vi "BMcalculate_v2_1.vi"() -> ()   [LabVIEW 2014]
uses:
  <vilib>/Analysis/NI_AALBase.lvlib
  <vilib>/Analysis/baseanly.llb/Mean (DBL).vi
  <vilib>/Analysis/NI_AALPro.lvlib
  <vilib>/Utility/file.llb/Write To Spreadsheet File (DBL).vi
  <vilib>/Utility/file.llb/Read From Spreadsheet File (string).vi
  <vilib>/Analysis/coordinate.llb/2D Cartesian Coordinate Rotation (Array).vi
panel:
  out "path out":path
  in  "(T=X , F=Y)":bool=TRUE
  in  "Filter window size":i32=100
  out "Array":dbl[](array[numeric])
  out "created path 2":path
  out "created path":path
  in  "Save Time-trace":bool
  in  "nm/pixel":dbl=72.5 format="%#_13g"
  in  "Folder path":path
  in  "?":bool
  in  "to":dbl=1.15 format="%#_13g"
  in  "x/y for all":dbl=0.85 format="%#_13g"
  out "filename":string
  in  "Filter mode":T1(ring)=enum."Median_slide window"
  in  "Save to vertical data ?":bool
  in  "?":enum32{"slide by slide", "delay"}(tab)=enum."delay"
  in  "?":bool
  in  "seconds to wait":u32
  in  "?":dbl=7.963 format="%#_13g"
  in  "?":dbl=48.61 format="%#_13g"
  in  "Save BM":bool
  in  "?":bool=TRUE
  in  "Save X-Y plot":bool
  in  "less than":dbl=0.2 format="%#_13g"
  in  "?":bool
  in  "?":bool
  in  "?":bool=TRUE
  in  "?":T2(tab)
  out "Filenames":string[](array[string])
  out "useful AOIs":i32[](array[numeric])
  out "# of AOI":i32[](array[numeric])
  out "% of useful AOIs":dbl
  out "tt # of AOIs":i32
  out "# of Frames":dbl[](array[numeric])
  out "tt # 0f useful AOIs":i32
  out "?":T3(graph)
  out "size(s)":i32
  out "X-Y plot":cluster{dbl[], dbl[]}(graph)
  out "Xstd":dbl
  out "ystd":dbl[](array[numeric])
  out "X":dbl format="%0.2f"
  out "Y":dbl format="%0.2f"
  out "?":T3(graph)
  out "tt # of useful AOIs":i32
  out "xstd":dbl[](array[numeric])
  out "# of AOI":i32
  out "y 2":dbl[](array[numeric])
  out "# of frames":dbl
  out "all y position (pixel)":dbl[][](array[numeric])
  out "all x position (pixel)":dbl[][](array[numeric])
  out "y":dbl[](array[numeric])
  out "x":dbl[](array[numeric])
  out "y":dbl[](array[numeric])
  out "x":dbl[](array[numeric])
  out "number":dbl[][](array[numeric])
  out "all rows":string[][](array[string])
  out "Useful aoi number":string[][](array[string])
  in  "Tab Control":enum32{"Time trace"}(tab)
  out "Time trace":T4(graph)
  in  "Highlight":dbl=30.0
  in  "±":dbl=30.0
  out "aoi":string
  in  "stop frame1":dbl
  in  "start frame1":dbl
  in  "start frame3":dbl
  in  "stop frame2":dbl
  in  "stop frame3":dbl
  in  "start frame2":dbl
  # "Critiria"
  # "±"
  # "nm"
  # "for ssDNA strande exchange \n                    23.776±6.613 nm"
  # "for D-loop  (90+4)\n                    48.61±7.963 nm"
  # "for D-loop  (150+4)\n                    49.57±8.56 nm"
  # "nm"
  # "Buffer wash"
  # "to"
  # "to"
  # "to"
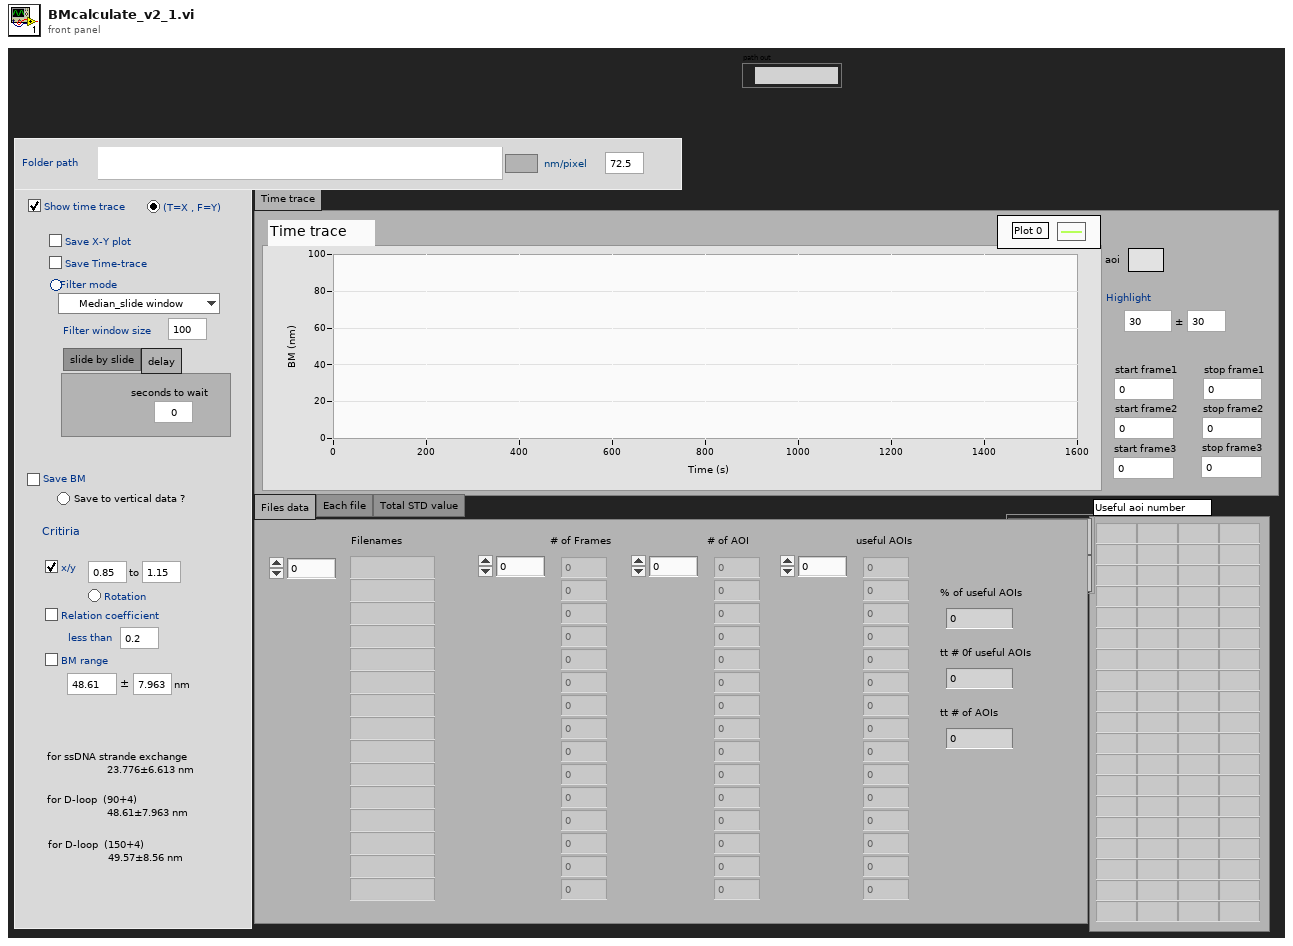
[diagram p1: front panel]
types:
  T1 = enum16{"Median_fix window", "Average_fix window", "Median_slide window", "Average_slide window"}
  T2 = enum32{"Files data", "Each file", "Total STD value"}
  T3 = cluster{"X Values":dbl[], "Histogram: h(x)":i32[]}
  T4 = cluster{"Filtered X":dbl[], "Filtered X":dbl[]}[]
  T5 = cluster{"all y position (pixel)":dbl[], "all x position (pixel)":dbl[]}
  T6 = cluster{"all x position (pixel)":dbl[], "all y position (pixel)":dbl[]}
  T7 = typedef "imagedata.ctl" = cluster{"image type":i32, "image depth":i32, "image":u8[], "mask":u8[], "colors":u32[], "Rectangle":cluster{"left":i16, "top":i16, "right":i16, "bottom":i16}}
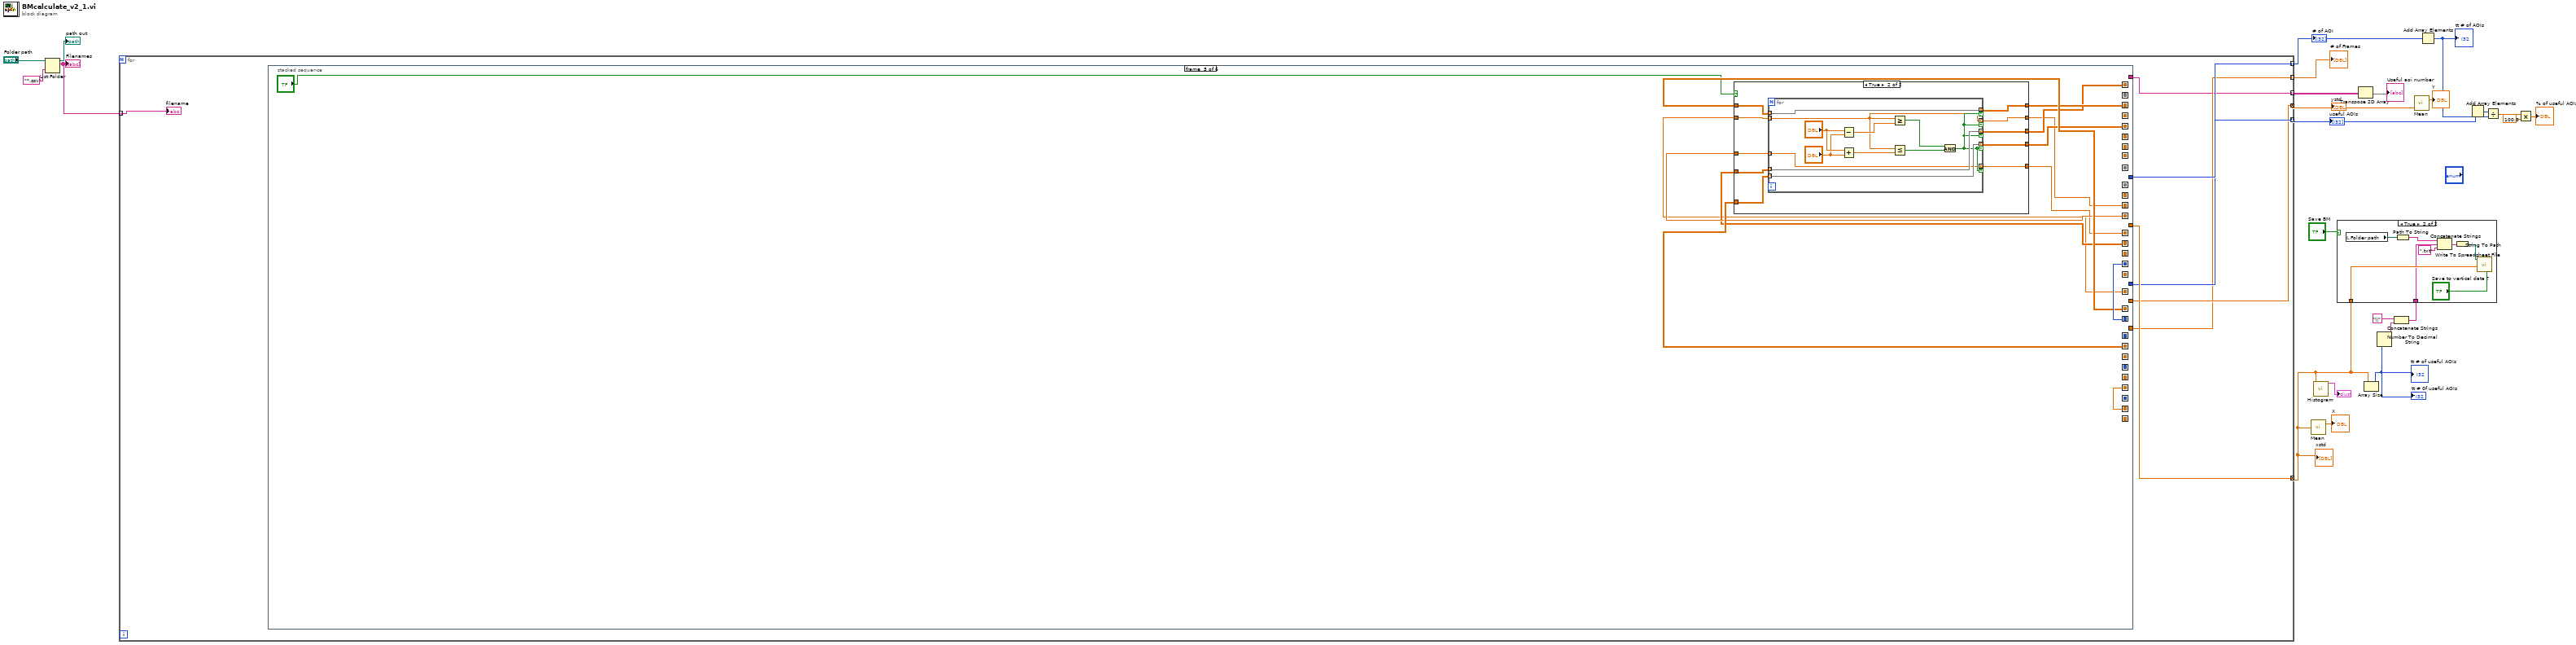
[diagram p0: block diagram]
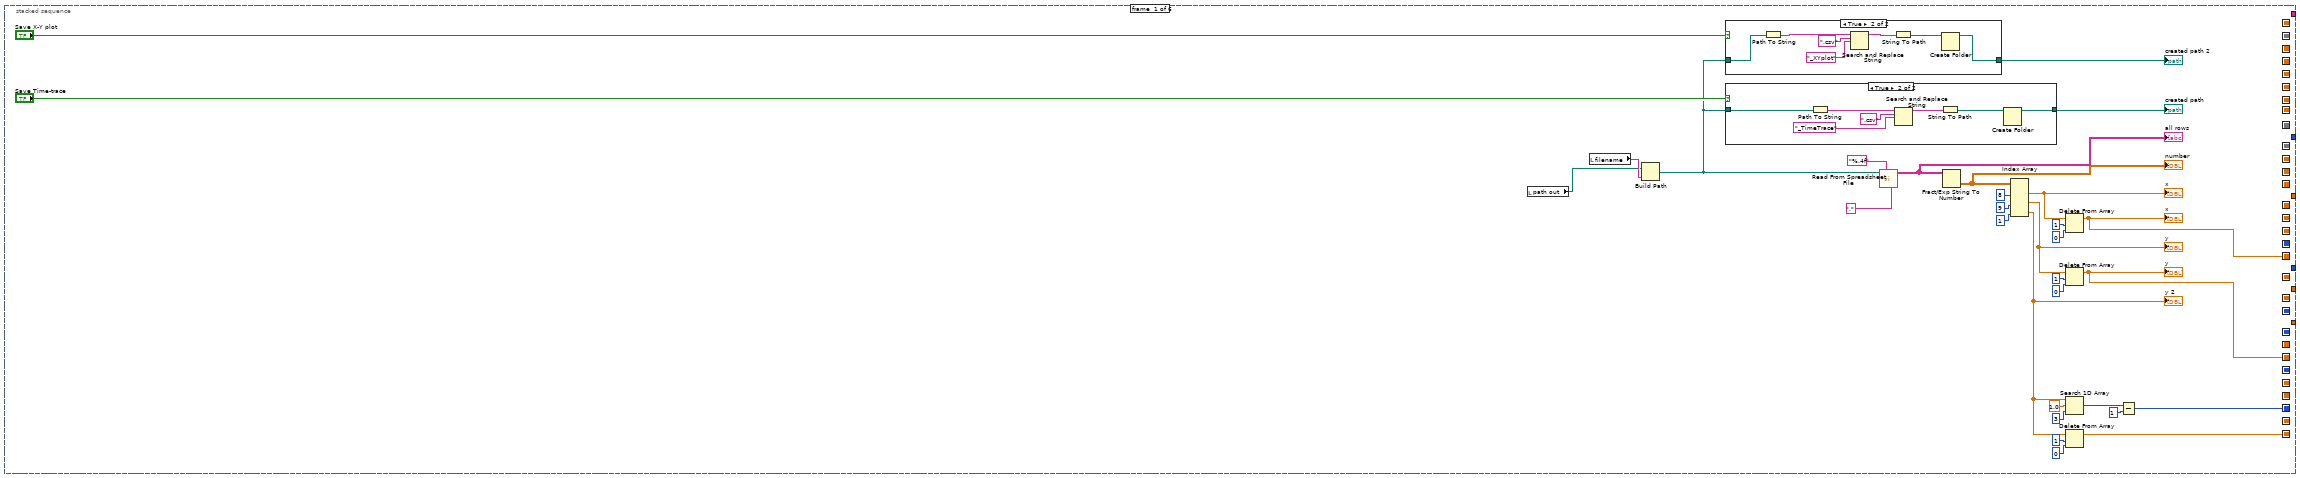
[diagram p3: hidden frame]
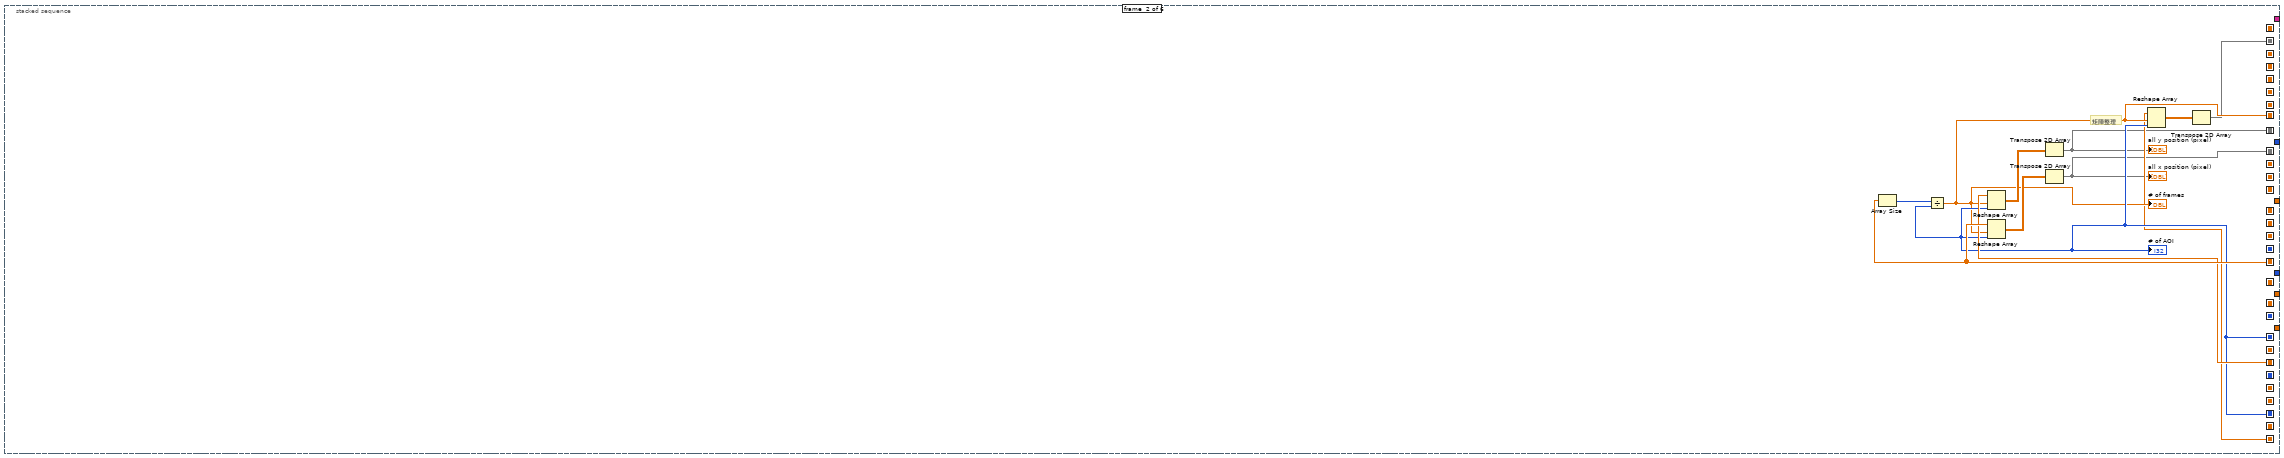
[diagram p6: hidden frame]
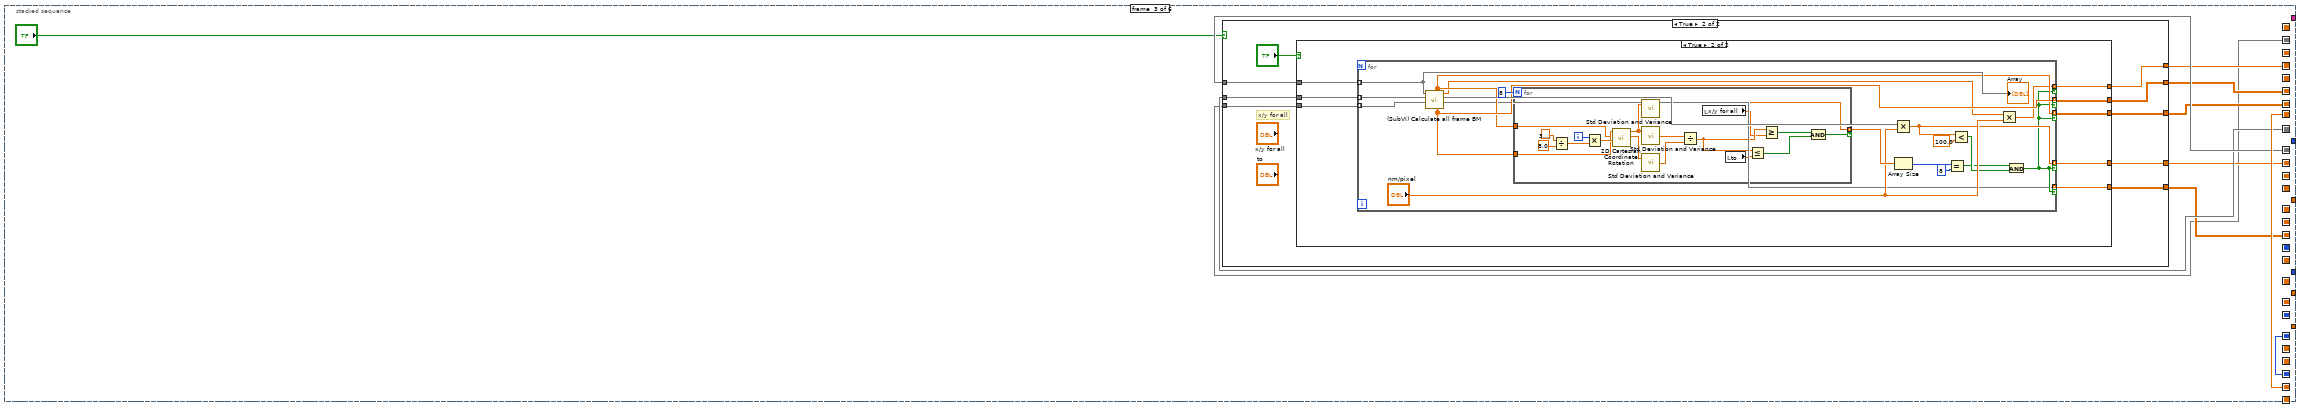
[diagram p7: hidden frame]
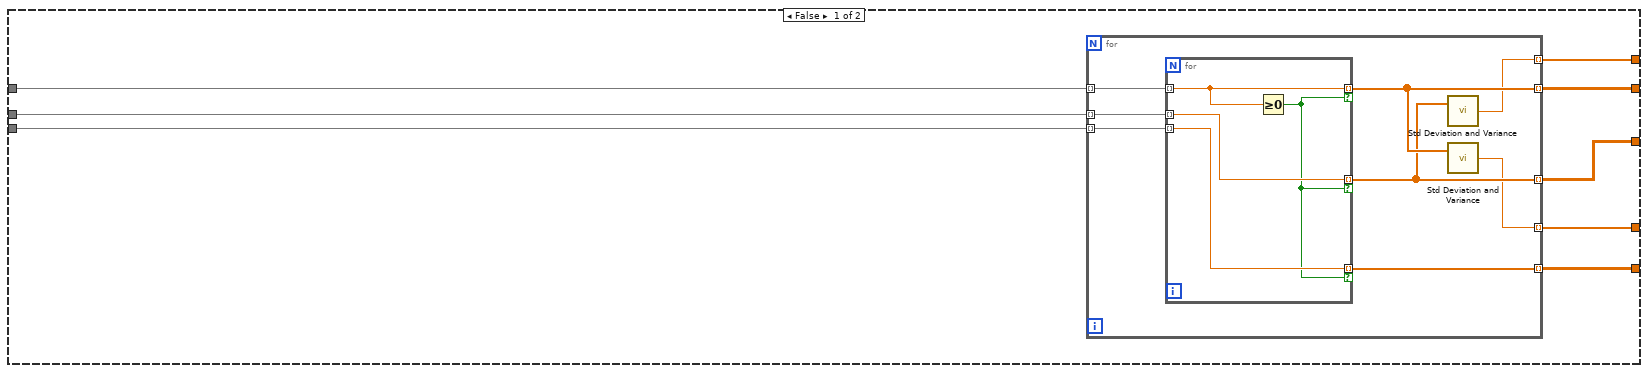
[diagram p8: hidden frame]
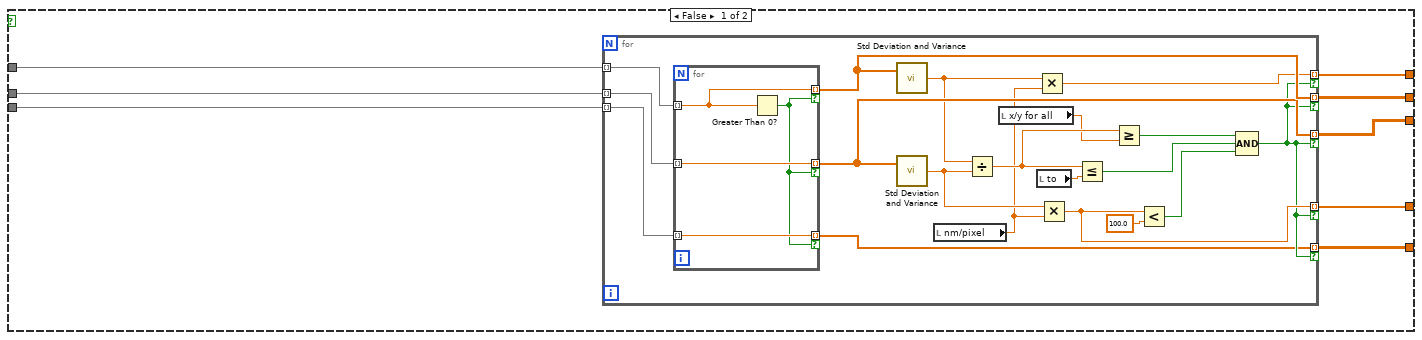
[diagram p9: hidden frame]
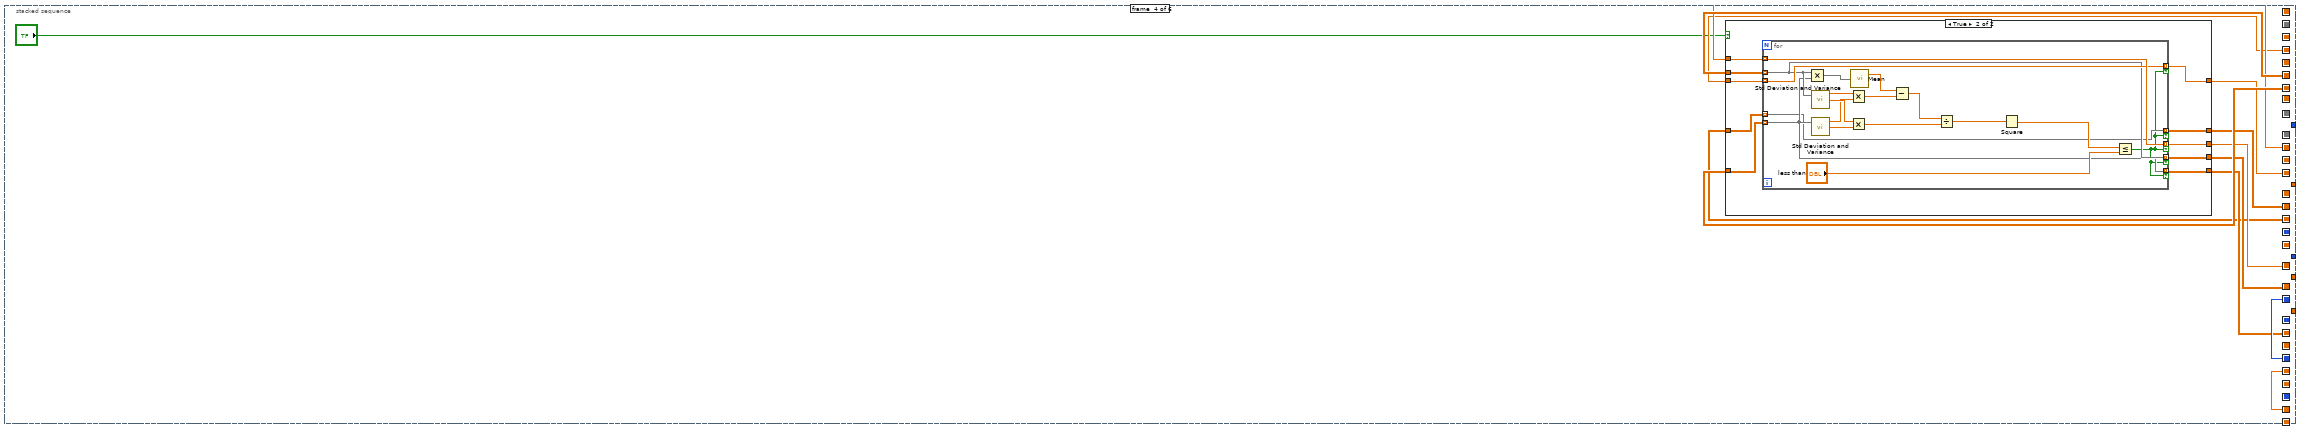
[diagram p10: hidden frame]
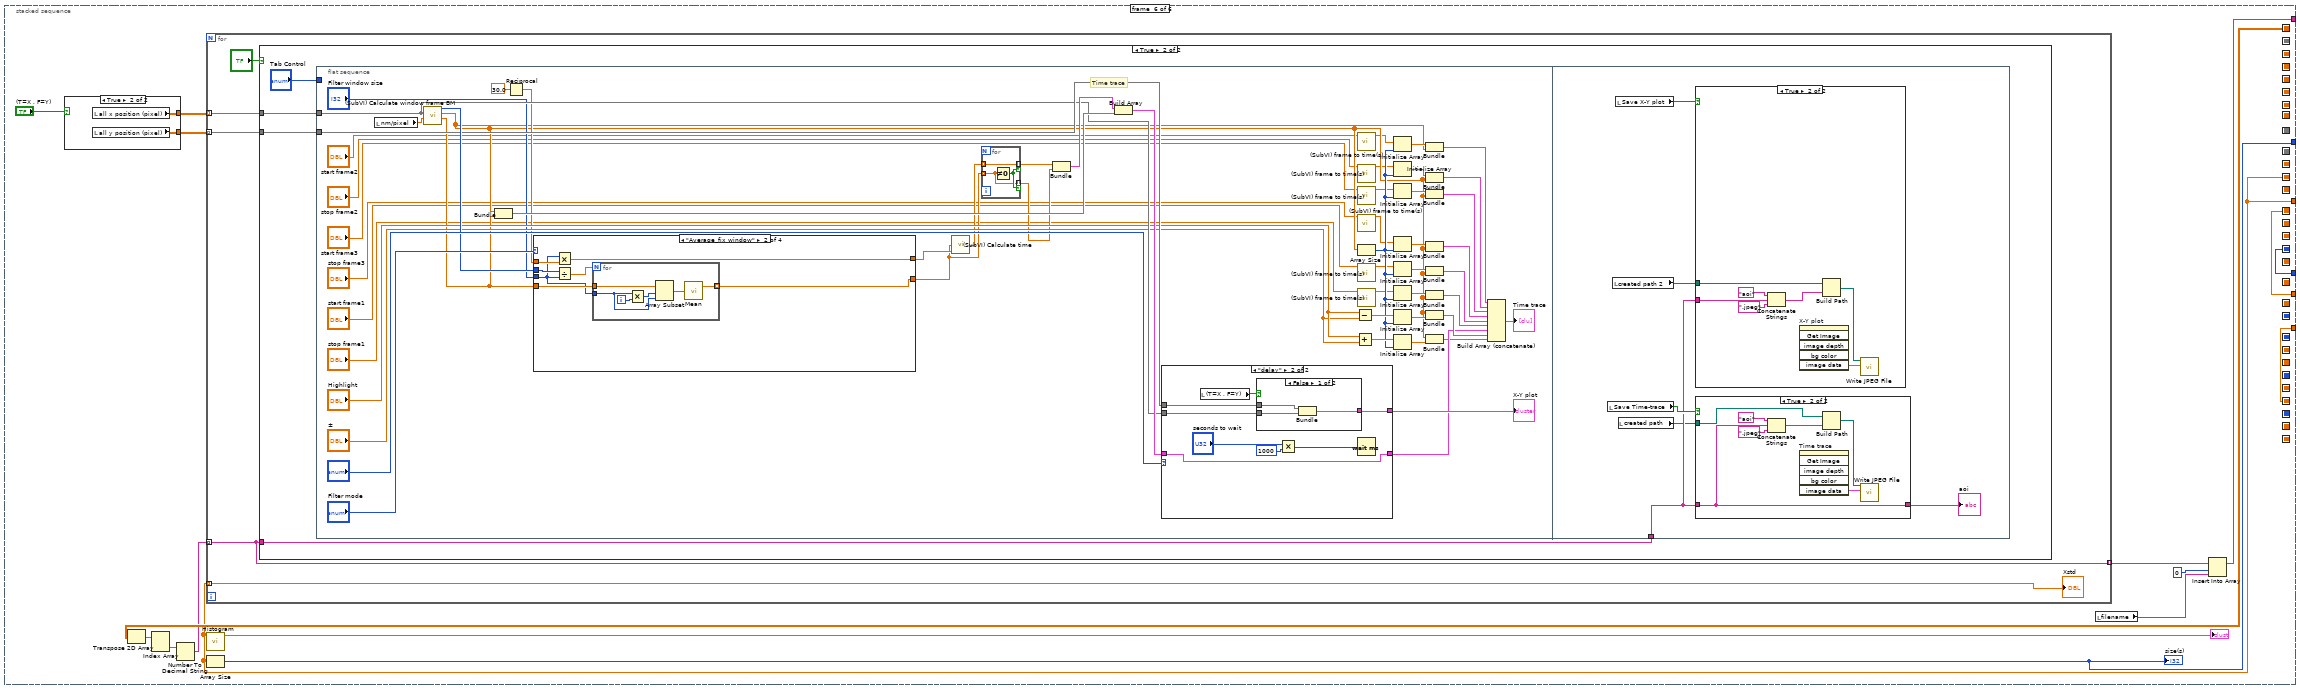
[diagram p13: hidden frame]
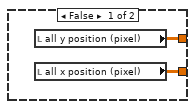
[diagram p14: hidden frame]
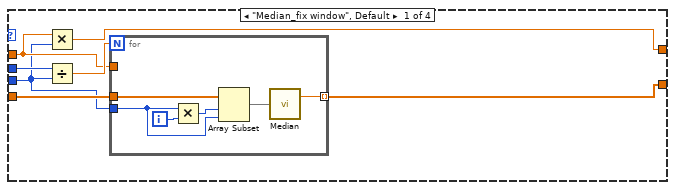
[diagram p16: hidden frame]
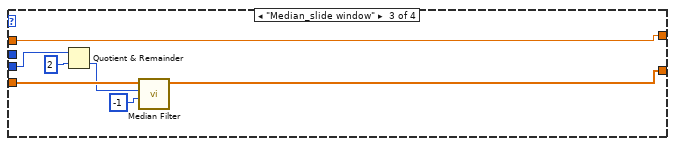
[diagram p17: hidden frame]
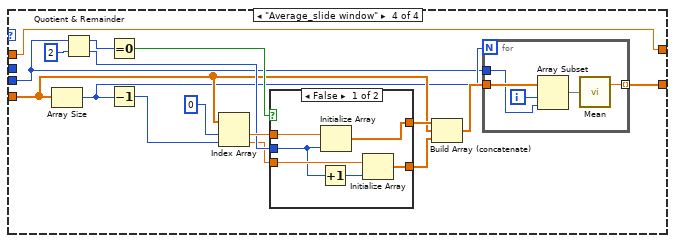
[diagram p18: hidden frame]
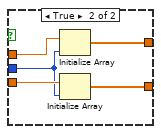
[diagram p19: hidden frame]
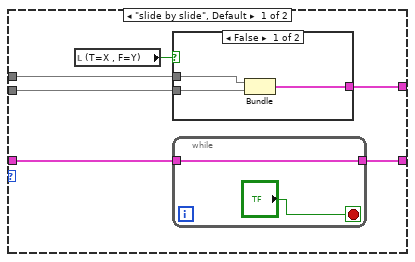
[diagram p20: hidden frame]
diagram:
  n1 = List Folder(path="Folder path", pattern="*.csv") -> (path out=→"path out":path, filenames=w1:string[])  [unwired: 2 in, 2 out]
  "Filenames" <- w1
  n2 = for {
    tunnel: [w31] -> w2 mode=concatenating
    tunnel: [w30] -> w21 mode=indexing
    tunnel: [w29] -> w20 mode=indexing
    tunnel: [w28] -> w12 mode=concatenating
    tunnel: [w27] -> w13 mode=indexing
    tunnel: [w26] -> w4 mode=indexing
    tunnel: w1 -> [w25] mode=indexing
    n3 = stacked-sequence {
      seq-local: [w51 _ _ _ _ _] -> [_ w87 _ _ _ _]
      seq-local: [w50 _ _ _ _ _] -> [_ w86 _ _ _ _]
      seq-local: [w44 _ _ _ _ _] -> [_ w85 _ _ _ _]
      seq-local: [w40 _ _ _ _ _] -> [_ w83 _ _ _ _]
      seq-local: [_ w84 _ _ _ _] -> [_ _ w101 _ _ _]
      seq-local: [_ w85 _ _ _ _] -> [_ _ w100 _ _ _]
      seq-local: [_ w80 _ _ _ _] -> [_ _ w99 _ _ _]
      seq-local: [_ w79 _ _ _ _] -> [_ _ w98 _ _ _]
      seq-local: [_ w81 _ _ _ _] -> [_ _ w91 _ _ _]
      seq-local: [_ _ w100 _ _ _] -> [_ _ _ w219 _ _]
      seq-local: [_ _ w101 _ _ _] -> [_ _ _ w218 _ _]
      seq-local: [_ _ w96 _ _ _] -> [_ _ _ w214 _ _]
      seq-local: [_ _ w95 _ _ _] -> [_ _ _ w217 _ _]
      seq-local: [_ _ w94 _ _ _] -> [_ _ _ w216 _ _]
      seq-local: [_ _ w93 _ _ _] -> [_ _ _ w215 _ _]
      seq-local: [_ _ w92 _ _ _] -> [_ _ _ w208 _ _]
      seq-local: [_ _ _ w219 _ _] -> [_ _ _ _ w265 _]
      seq-local: [_ _ _ w218 _ _] -> [_ _ _ _ w264 _]
      seq-local: [_ _ _ w209 _ _] -> [_ _ _ _ w259 _]
      seq-local: [_ _ _ w212 _ _] -> [_ _ _ _ w263 _]
      seq-local: [_ _ _ w211 _ _] -> [_ _ _ _ w261 _]
      seq-local: [_ _ _ w210 _ _] -> [_ _ _ _ w254 _]
      seq-local: [_ _ _ w207 _ _] -> [_ _ _ _ w256 _]
      seq-local: [_ _ _ _ w265 _] -> [_ _ _ _ _ w311]
      seq-local: [_ _ _ _ w264 _] -> [_ _ _ _ _ w310]
      seq-local: [_ _ _ _ w258 _] -> [_ _ _ _ _ w309]
      seq-local: [_ _ _ _ w262 _] -> [_ _ _ _ _ _]
      seq-local: [_ _ _ _ w260 _] -> [_ _ _ _ _ _]
      seq-local: [_ _ _ _ w253 _] -> [_ _ _ _ _ w302]
      seq-local: [_ _ _ _ w255 _] -> [_ _ _ _ _ w306]
      tunnel: [_ _ _ _ _ w302] -> w31
      tunnel: [_ _ _ _ _ w307] -> w30
      tunnel: [_ _ _ _ _ w311] -> w29
      tunnel: [_ _ _ _ _ w310] -> w27
      tunnel: [_ _ _ _ _ w309] -> w28
      tunnel: [_ _ _ _ _ w298] -> w26
      frame #0 {
        n4 = local read "path out"() -> (w32:path)
        n5 = local read "filename"() -> (w33:string)
        n6 = Build Path(base path=w32, name or relative path=w33) -> (appended path=w35:path)
        n7 = case shown="True" "Save X-Y plot" {
          tunnel: w35 -> [w71 w78]
          tunnel: [w71 w72] -> w39
          frame False {
          }
          frame True {
            n8 = Path To String(path=w78) -> (string=w77:string)
            n9 = Search and Replace String(input string=w77, search string=".csv", replace string="_XYplot" ("replace string (\"\")")) -> (result string=w74:string)  [unwired: 5 in, 3 out]
            n10 = String To Path(string=w74) -> (path=w73:path)
            n11 = Create Folder(path (use dialog)=w73) -> (created path=w72:path)  [unwired: 2 in, 2 out]
          }
        }
        "created path 2" <- w39
        n12 = case shown="True" "Save Time-trace" {
          tunnel: w35 -> [w63 w70]
          tunnel: [w63 w64] -> w34
          frame False {
          }
          frame True {
            n13 = Path To String(path=w70) -> (string=w69:string)
            n14 = Search and Replace String(input string=w69, search string=".csv", replace string="_TimeTrace" ("replace string (\"\")")) -> (result string=w66:string)  [unwired: 5 in, 3 out]
            n15 = String To Path(string=w66) -> (path=w65:path)
            n16 = Create Folder(path (use dialog)=w65) -> (created path=w64:path)  [unwired: 2 in, 2 out]
          }
        }
        "created path" <- w34
        n17 = call-poly <vilib>:"Read From Spreadsheet File.vi"("delimiter (\\t)"="," ("delimiter (\\t)"), "format (%s)"="%.4f" ("format (%.3f)"), "file path (dialog if empty)"=w35) -> ("all rows"=w61:string[][])  [unwired: 4 in, 4 out]
        "all rows" <- w61
        n18 = Fract/Exp String To Number(string=w61) -> (number=w60:dbl[][])  [unwired: 3 in, 1 out]
        "number" <- w60
        n19 = Index Array(array=w60, index (col) #1=8 ("disabled index (col)"), index (col) #2=9 ("index (col)"), index (col) #3=1 ("index (col)")) -> (element #1=w52:dbl[], element #2=w53:dbl[], element #3=w41:dbl[])  [unwired: 3 in]
        "x" <- w52
        "y" <- w53
        "y 2" <- w41
        n20 = Delete From Array(array=w52, length=1, index=0) -> (array with subset deleted=w51:dbl[])  [unwired: 1 out]
        "x" <- w51
        n21 = Delete From Array(array=w53, length=1, index=0) -> (array with subset deleted=w50:dbl[])  [unwired: 1 out]
        "y" <- w50
        n22 = Search 1D Array(1D array=w41, element=1.0, start index (0)=3) -> (index of element=w46:i32)
        n23 = Delete From Array(array=w41, length=1, index=0) -> (array with subset deleted=w40:dbl[])  [unwired: 1 out]
        n24 = Subtract(x=w46, y=1) -> (x-y=w44:i32)
      }
      frame #1 {
        # "矩陣整理"
        n25 = Array Size(array=w87) -> (size(s)=w88:i32)
        n26 = Divide(x=w88, y=w85) -> (x/y=w84:dbl)
        "# of frames" <- w84
        n27 = Reshape Array(w86, w84, w85) -> (w90:dbl[][])
        n28 = Reshape Array(w87, w84, w85) -> (w89:dbl[][])
        n29 = Transpose 2D Array(2D array=w90) -> (transposed array=w79:dbl[][])
        "all y position (pixel)" <- w79
        n30 = Transpose 2D Array(2D array=w89) -> (transposed array=w80:dbl[][])
        "all x position (pixel)" <- w80
        n31 = Reshape Array(w83, w84, w85) -> (w82:dbl[][])
        n32 = Transpose 2D Array(2D array=w82) -> (transposed array=w81:dbl[][])
        "# of AOI" <- w85
      }
      frame #2 {
        n33 = case shown="True" "?" {
          tunnel: [w107 w130] -> w95
          tunnel: [w106 w129] -> w94
          tunnel: w99 -> [w109 w128]
          tunnel: w98 -> [w108 w127]
          tunnel: [w105 w126] -> w93
          tunnel: [w104 w125] -> w96
          tunnel: w91 -> [w103 w123]
          tunnel: [w102 w122] -> w92
          frame False {
            n34 = for {
              tunnel: w109 -> [w117] mode=indexing
              tunnel: w108 -> [w116] mode=indexing
              tunnel: [w115] -> w107 mode=indexing
              tunnel: [w114] -> w106 mode=indexing
              tunnel: [w113] -> w105 mode=indexing
              tunnel: [w112] -> w104 mode=indexing
              tunnel: w103 -> [w111] mode=indexing
              tunnel: [w110] -> w102 mode=indexing
              n35 = for {
                tunnel: w117 -> [w120] mode=indexing
                tunnel: w116 -> [w121] mode=indexing
                tunnel: [w120] -> w115 mode=indexing if=w118
                tunnel: [w121] -> w114 mode=indexing if=w118
                tunnel: w111 -> [w119] mode=indexing
                tunnel: [w119] -> w110 mode=indexing if=w118
                n36 = Greater Or Equal To 0?(x=w120) -> (x >= 0?=w118:bool)
              }
              n37 = call <vilib>:"Std Deviation and Variance.vi"("X"=w114) -> ("standard deviation"=w112:dbl)  [unwired: 1 in, 2 out]
              n38 = call <vilib>:"Std Deviation and Variance.vi"("X"=w115) -> ("standard deviation"=w113:dbl)  [unwired: 1 in, 2 out]
            }
          }
          frame True {
            # "x/y for all"
            n39 = case shown="True" "?" {
              tunnel: w127 -> [w137 w169]
              tunnel: w128 -> [w138 w168]
              tunnel: [w136 w167] -> w130
              tunnel: [w135 w166] -> w129
              tunnel: [w134 w165] -> w126
              tunnel: [w133 w164] -> w125
              tunnel: w123 -> [w132 w163]
              tunnel: [w131 w162] -> w122
              frame False {
                n40 = for {
                  tunnel: w138 -> [w157] mode=indexing
                  tunnel: w137 -> [w156] mode=indexing
                  tunnel: [w155] -> w136 mode=indexing if=w142
                  tunnel: [w154] -> w135 mode=indexing if=w142
                  tunnel: [w143] -> w134 mode=indexing if=w142
                  tunnel: [w146] -> w133 mode=indexing if=w142
                  tunnel: [w140] -> w131 mode=indexing if=w142
                  tunnel: w132 -> [w141] mode=indexing
                  n41 = for {
                    tunnel: w157 -> [w160] mode=indexing
                    tunnel: w156 -> [w161] mode=indexing
                    tunnel: [w160] -> w155 mode=indexing if=w158
                    tunnel: [w161] -> w154 mode=indexing if=w158
                    tunnel: w141 -> [w159] mode=indexing
                    tunnel: [w159] -> w140 mode=indexing if=w158
                    n42 = Greater Than 0?(x=w160) -> (x > 0?=w158:bool)
                  }
                  n43 = call <vilib>:"Std Deviation and Variance.vi"("X"=w155) -> ("standard deviation"=w147:dbl)  [unwired: 1 in, 2 out]
                  n44 = call <vilib>:"Std Deviation and Variance.vi"("X"=w154) -> ("standard deviation"=w148:dbl)  [unwired: 1 in, 2 out]
                  n45 = local read "nm/pixel"() -> (w139:dbl)
                  n46 = Divide(x=w147, y=w148) -> (x/y=w153:dbl)
                  n47 = local read "x/y for all"() -> (w152:dbl)
                  n48 = Multiply(x=w147, y=w139) -> (x*y=w146:dbl)
                  n49 = local read "to"() -> (w151:dbl)
                  n50 = Multiply(x=w148, y=w139) -> (x*y=w143:dbl)
                  n51 = Less Or Equal?(x=w153, y=w151) -> (x <= y?=w149:bool)
                  n52 = Greater Or Equal?(x=w153, y=w152) -> (x >= y?=w150:bool)
                  n53 = Less?(x=w143, y=100.0) -> (x < y?=w144:bool)
                  n54 = Compound Arithmetic op=AND(w150, w149, w144) -> (w142:bool)
                }
              }
              frame True {
                n55 = for {
                  tunnel: w168 -> [w188] mode=indexing
                  tunnel: w169 -> [w187] mode=indexing
                  tunnel: [w173] -> w165 mode=indexing if=w172
                  tunnel: [w180] -> w166 mode=indexing if=w172
                  tunnel: [w181] -> w167 mode=indexing if=w172
                  tunnel: [w178] -> w164 mode=indexing if=w172
                  tunnel: [w171] -> w162 mode=indexing if=w172
                  tunnel: w163 -> [w170] mode=indexing
                  n56 = call "(SubVI) Calculate all frame BM.vi"(9:w170, "y position (pixel)"=w187, "x position (pixel)"=w188) -> (1:w171, 2:w182, "x standard deviation"=w179:dbl, "y position (delete y fit error)"=w181:dbl[], "x position (delete x fit error)"=w180:dbl[])  [unwired: 3 in, 1 out]
                  n57 = for {
                    N: 8 -> [_]
                    tunnel: w181 -> [w201]
                    tunnel: w180 -> [w200]
                    tunnel: [w192] -> w183 mode=indexing if=w191
                    i -> [w202]
                    n58 = Divide(x=3.141592653589793, y=8.0) -> (x/y=w205:dbl)
                    n59 = Multiply(x=w202, y=w205) -> (x*y=w203:dbl)
                    n60 = call-poly <vilib>:"2D Cartesian Coordinate Rotation.vi"("theta"=w203, "Y"=w200, "X"=w201) -> ("Y Out"=w193:dbl[], "X Out"=w194:dbl[])  [unwired: 6 in, 1 out]
                    n61 = call <vilib>:"Std Deviation and Variance.vi"("X"=w194) -> ("mean"=w192:dbl)  [unwired: 1 in, 2 out]
                    n62 = call <vilib>:"Std Deviation and Variance.vi"("X"=w194) -> ("standard deviation"=w199:dbl)  [unwired: 1 in, 2 out]
                    n63 = call <vilib>:"Std Deviation and Variance.vi"("X"=w193) -> ("standard deviation"=w198:dbl)  [unwired: 1 in, 2 out]
                    n64 = Divide(x=w199, y=w198) -> (x/y=w197:dbl)
                    n65 = local read "x/y for all"() -> (w190:dbl)
                    n66 = local read "to"() -> (w189:dbl)
                    n67 = Less Or Equal?(x=w197, y=w189) -> (x <= y?=w195:bool)
                    n68 = Greater Or Equal?(x=w197, y=w190) -> (x >= y?=w196:bool)
                    n69 = Compound Arithmetic op=AND(w196, w195) -> (w191:bool)
                  }
                  n70 = Multiply(x=w182, y="nm/pixel") -> (x*y=w173:dbl)
                  n71 = Array Size(array=w183) -> (size(s)=w185:i32)
                  n72 = Equal?(x=w185, y=8) -> (x = y?=w174:bool)
                  n73 = Less?(x=w173, y=100.0) -> (x < y?=w175:bool)
                  n74 = Multiply(x=w179, y="nm/pixel") -> (x*y=w178:dbl)
                  n75 = Compound Arithmetic op=AND(w174, w175) -> (w172:bool)
                  "Array" <- w188
                }
              }
            }
          }
        }
      }
      frame #3 {
        n76 = case shown="True" "?" {
          tunnel: w217 -> [w224 w234]
          tunnel: w216 -> [w223 w233]
          tunnel: w215 -> [w222 w230]
          tunnel: w214 -> [w221 w228]
          tunnel: [w224 w232] -> w212
          tunnel: [w223 w231] -> w211
          tunnel: [w222 w229] -> w210
          tunnel: [w221 w227] -> w209
          tunnel: w208 -> [w220 w226]
          tunnel: [w220 w225] -> w207
          frame False {
          }
          frame True {
            n77 = for {
              tunnel: w234 -> [w240] mode=indexing
              tunnel: w233 -> [w239] mode=indexing
              tunnel: [w240] -> w232 mode=indexing if=w235
              tunnel: [w239] -> w231 mode=indexing if=w235
              tunnel: [w247] -> w229 mode=indexing if=w235
              tunnel: w230 -> [w247] mode=indexing
              tunnel: w228 -> [w246] mode=indexing
              tunnel: [w246] -> w227 mode=indexing if=w235
              tunnel: [w236] -> w225 mode=indexing if=w235
              tunnel: w226 -> [w236] mode=indexing
              n78 = Multiply(x=w240, y=w239) -> (x*y=w238:dbl[])
              n79 = call <vilib>:"Std Deviation and Variance.vi"("X"=w240) -> ("mean"=w243:dbl, "standard deviation"=w245:dbl)  [unwired: 1 in, 1 out]
              n80 = call <vilib>:"Std Deviation and Variance.vi"("X"=w239) -> ("mean"=w242:dbl, "standard deviation"=w244:dbl)  [unwired: 1 in, 1 out]
              n81 = Multiply(x=w243, y=w242) -> (x*y=w241:dbl)
              n82 = Multiply(x=w245, y=w244) -> (x*y=w248:dbl)
              n83 = call-poly <vilib>:"Mean.vi"("X"=w238) -> ("mean"=w237:dbl)  [unwired: 1 out]
              n84 = Subtract(x=w237, y=w241) -> (x-y=w249:dbl)
              n85 = Divide(x=w249, y=w248) -> (x/y=w250:dbl)
              n86 = Square(x=w250) -> (x^2=w251:dbl)
              n87 = Less Or Equal?(x=w251, y="less than") -> (x <= y?=w235:bool)
            }
          }
        }
      }
      frame #4 {
        n88 = case shown="True" "?" {
          tunnel: [w271 w281] -> w262
          tunnel: w263 -> [w271 w282]
          tunnel: w261 -> [w270 w280]
          tunnel: [w270 w279] -> w260
          tunnel: w254 -> [w269 w278]
          tunnel: [w269 w277] -> w253
          tunnel: w259 -> [w268 w276]
          tunnel: [w268 w275] -> w258
          tunnel: w256 -> [w267 w274]
          tunnel: [w266 w273] -> w255
          frame False {
            n89 = for {
              tunnel: w267 -> [w272] mode=indexing
              tunnel: [w272] -> w266 mode=indexing
            }
          }
          frame True {
            n90 = for {
              tunnel: [w294] -> w281 mode=indexing if=w289
              tunnel: w282 -> [w294] mode=indexing
              tunnel: [w293] -> w279 mode=indexing if=w289
              tunnel: w280 -> [w293] mode=indexing
              tunnel: [w283] -> w277 mode=indexing if=w289
              tunnel: w278 -> [w283] mode=indexing
              tunnel: w276 -> [w288] mode=indexing
              tunnel: [w288] -> w275 mode=indexing if=w289
              tunnel: [w290] -> w273 mode=indexing if=w289
              tunnel: w274 -> [w290] mode=indexing
              n91 = Subtract(x="?", y="?") -> (x-y=w285:dbl)
              n92 = Add(x="?", y="?") -> (x+y=w284:dbl)
              n93 = Greater Or Equal?(x=w283, y=w285) -> (x >= y?=w292:bool)
              n94 = Less Or Equal?(x=w283, y=w284) -> (x <= y?=w291:bool)
              n95 = Compound Arithmetic op=AND(w292, w291) -> (w289:bool)
            }
          }
        }
      }
      frame #5 {
        n96 = case shown="True" "(T=X , F=Y)" {
          tunnel: [w313 w315] -> w296
          tunnel: [w312 w314] -> w295
          frame False {
            n97 = local read "all y position (pixel)"() -> (w313:dbl[][])
            n98 = local read "all x position (pixel)"() -> (w312:dbl[][])
          }
          frame True {
            n99 = local read "all x position (pixel)"() -> (w315:dbl[][])
            n100 = local read "all y position (pixel)"() -> (w314:dbl[][])
          }
        }
        n101 = Transpose 2D Array(2D array=w306) -> (transposed array=w305:dbl[][])
        n102 = Index Array(array=w305) -> (element=w304:dbl[])  [unwired: 2 in]
        n103 = Number To Decimal String(number=w304) -> (decimal integer string=w303:string[])  [unwired: 1 in]
        n104 = for {
          tunnel: w296 -> [w319] mode=indexing
          tunnel: w295 -> [w320] mode=indexing
          tunnel: w303 -> [w316] mode=indexing
          tunnel: w302 -> [w317] mode=indexing
          tunnel: [w316] -> w299 mode=indexing
          n105 = case shown="True" "?" {
            tunnel: w320 -> [_ w324]
            tunnel: w319 -> [_ w323]
            tunnel: w316 -> [_ w322]
            frame False {
            }
            frame True {
              n106 = flat-sequence {
                tunnel: w324 -> [w370]
                tunnel: w323 -> [w369]
                tunnel: "Tab Control" -> [_]
                tunnel: w322 -> [w480]
                frame #0 {
                  # "Time trace"
                  n107 = local read "nm/pixel"() -> (w359:dbl)
                  n108 = call "(SubVI) Calculate window frame BM.vi"("nm/pixel"=w359, "all x position (pixel)"=w369) -> ("BM"=w354:dbl[], "sec"=w341:dbl[], "frame"=w375:i32)  [unwired: 3 in]
                  n109 = Bundle("sec"=w341, "BM"=w354) -> (w374:cluster{"sec":dbl[], "BM":dbl[]})  [unwired: 1 in]
                  n110 = Reciprocal(x=30.0) -> (1/x=w356:dbl)
                  n111 = case shown="\"Average_fix window\"" "Filter mode" {
                    tunnel: [w388 w399 w414 w431] -> w353
                    tunnel: w354 -> [w389 w400 w415 w420]
                    tunnel: w375 -> [w387 w402 _ _]
                    tunnel: "Filter window size" -> [w383 w396 w411 w417]
                    tunnel: w356 -> [w385 w398 w413 w416]
                    tunnel: [w384 w397 w413 w416] -> w355
                    frame "Median_fix window", Default {
                      n112 = Multiply(x=w385, y=w383) -> (x*y=w384:dbl)
                      n113 = Divide(x=w387, y=w383) -> (x/y=w386:dbl)
                      n114 = for {
                        N: w386 -> [_]
                        tunnel: w389 -> [w395]
                        tunnel: [w393] -> w388 mode=indexing
                        tunnel: w383 -> [w390]
                        tunnel: w385 -> [_]
                        i -> [w392]
                        n115 = Multiply(x=w390, y=w392) -> (x*y=w391:i32)
                        n116 = Array Subset(array=w395, index=w391, length=w390) -> (w394:dbl[])
                        n117 = call <vilib>:"Median.vi"("X"=w394) -> ("median"=w393:dbl)  [unwired: 1 out]
                      }
                    }
                    frame "Average_fix window" {
                      n118 = Multiply(x=w396, y=w398) -> (x*y=w397:dbl)
                      n119 = Divide(x=w402, y=w396) -> (x/y=w401:dbl)
                      n120 = for {
                        N: w401 -> [_]
                        tunnel: w400 -> [w408]
                        tunnel: [w406] -> w399 mode=indexing
                        tunnel: w396 -> [w404]
                        i -> [w405]
                        n121 = Multiply(x=w404, y=w405) -> (x*y=w403:i32)
                        n122 = Array Subset(array=w408, index=w403, length=w404) -> (w407:dbl[])
                        n123 = call-poly <vilib>:"Mean.vi"("X"=w407) -> ("mean"=w406:dbl)  [unwired: 1 out]
                      }
                    }
                    frame "Median_slide window" {
                      n124 = Quotient & Remainder(x=w411, y=2) -> (floor(x/y)=w409:i32)  [unwired: 1 out]
                      n125 = call <vilib>:"Median Filter.vi"("right rank"=-1, "left rank"=w409, "X"=w415) -> ("Filtered X"=w414:dbl[])  [unwired: 7 in, 1 out]
                    }
                    frame "Average_slide window" {
                      n126 = Array Size(array=w420) -> (size(s)=w418:i32)
                      n127 = Quotient & Remainder(x=w417, y=2) -> (x-y*floor(x/y)=w427:i32, floor(x/y)=w425:i32)
                      n128 = Equal To 0?(x=w427) -> (x = 0?=w426:bool)
                      n129 = Decrement(x=w418) -> (x-1=w424:i32)
                      n130 = Index Array(array=w420, index #1=0 ("index"), index #2=w424) -> (element #1=w429:dbl, element #2=w423:dbl)
                      n131 = case shown="False" w426 {
                        tunnel: w429 -> [w437 w442]
                        tunnel: w425 -> [w434 w440]
                        tunnel: w423 -> [w436 w441]
                        tunnel: [w432 w439] -> w422
                        tunnel: [w433 w438] -> w421
                        frame False {
                          n132 = Increment(x=w434) -> (x+1=w435:i32)
                          n133 = Initialize Array(w437, w434) -> (w432:dbl[])
                          n134 = Initialize Array(w436, w435) -> (w433:dbl[])
                        }
                        frame True {
                          n135 = Initialize Array(w442, w440) -> (w439:dbl[])
                          n136 = Initialize Array(w441, w440) -> (w438:dbl[])
                        }
                      }
                      n137 = Build Array (concatenate)(w422, w420, w421) -> (w419:dbl[])
                      n138 = for {
                        N: w418 -> [_]
                        tunnel: w419 -> [w447]
                        tunnel: [w445] -> w431 mode=indexing
                        tunnel: w417 -> [w443]
                        i -> [w444]
                        n139 = Array Subset(array=w447, index=w444, length=w443) -> (w446:dbl[])
                        n140 = call-poly <vilib>:"Mean.vi"("X"=w446) -> ("mean"=w445:dbl)  [unwired: 1 out]
                      }
                    }
                  }
                  n141 = call "(SubVI) Calculate time.vi"("dt"=w355, "BM"=w353) -> ("Time (s)"=w352:dbl[])  [unwired: 3 in]
                  n142 = for {
                    tunnel: w353 -> [w380] mode=indexing
                    tunnel: [w380] -> w350 mode=indexing if=w381
                    tunnel: w352 -> [w382] mode=indexing
                    tunnel: [w382] -> w351 mode=indexing if=w381
                    n143 = Not Equal To 0?(x=w380) -> (x != 0?=w381:bool)
                  }
                  n144 = Bundle(w351, w350) -> (w379:cluster{dbl[], dbl[]})  [unwired: 1 in]
                  n145 = Build Array(w379, w374) -> (w378:cluster{"sec":dbl[], "BM":dbl[]}[])
                  n146 = case shown="\"delay\"" "?" {
                    tunnel: w378 -> [w453 w469]
                    tunnel: [w452 w469] -> w371
                    tunnel: w369 -> [w451 w465]
                    tunnel: w370 -> [w450 w464]
                    tunnel: [w449 w463] -> w373
                    frame "slide by slide", Default {
                      n147 = local read "(T=X , F=Y)"() -> (w448:bool)
                      n148 = case shown="False" w448 {
                        tunnel: w451 -> [w456 w459]
                        tunnel: w450 -> [w455 w458]
                        tunnel: [w454 w457] -> w449
                        frame False {
                          n149 = Bundle("all y position (pixel)"=w455, "all x position (pixel)"=w456) -> (w454:T5)  [unwired: 1 in]
                        }
                        frame True {
                          n150 = Bundle("all x position (pixel)"=w459, "all y position (pixel)"=w458) -> (w457:T6)  [unwired: 1 in]
                        }
                      }
                      n151 = while {
                        tunnel: w453 -> [w460]
                        tunnel: [w460] -> w452
                        stop <- "?" stop-if-true
                      }
                    }
                    frame "delay" {
                      n152 = local read "(T=X , F=Y)"() -> (w462:bool)
                      n153 = case shown="False" w462 {
                        tunnel: w465 -> [w472 w475]
                        tunnel: w464 -> [w471 w474]
                        tunnel: [w470 w473] -> w463
                        frame False {
                          n154 = Bundle("all y position (pixel)"=w471, "all x position (pixel)"=w472) -> (w470:T5)  [unwired: 1 in]
                        }
                        frame True {
                          n155 = Bundle("all x position (pixel)"=w475, "all y position (pixel)"=w474) -> (w473:T6)  [unwired: 1 in]
                        }
                      }
                      n156 = Multiply(x="seconds to wait", y=u32 1000) -> (x*y=w467:u32)
                      n157 = Wait (ms)(milliseconds to wait=w467) -> ()  [unwired: 1 out]
                    }
                  }
                  "X-Y plot" <- w373
                  n158 = Subtract(x="Highlight", y="±") -> (x-y=w363:dbl)
                  n159 = Add(x="Highlight", y="±") -> (x+y=w362:dbl)
                  n160 = call "(SubVI) frame to time(s).vi"("Numeric in"="start frame2") -> ("Numeric out"=w330:dbl)  [unwired: 10 in]
                  n161 = call "(SubVI) frame to time(s).vi"("Numeric in"="stop frame2") -> ("Numeric out"=w329:dbl)  [unwired: 10 in]
                  n162 = call "(SubVI) frame to time(s).vi"("Numeric in"="start frame3") -> ("Numeric out"=w326:dbl)  [unwired: 10 in]
                  n163 = call "(SubVI) frame to time(s).vi"("Numeric in"="stop frame3") -> ("Numeric out"=w325:dbl)  [unwired: 10 in]
                  n164 = Array Size(array=w341) -> (size(s)=w347:i32)
                  n165 = call "(SubVI) frame to time(s).vi"("Numeric in"="start frame1") -> ("Numeric out"=w336:dbl)  [unwired: 10 in]
                  n166 = call "(SubVI) frame to time(s).vi"("Numeric in"="stop frame1") -> ("Numeric out"=w333:dbl)  [unwired: 10 in]
                  n167 = Initialize Array(w330, w347) -> (w345:dbl[])
                  n168 = Initialize Array(w329, w347) -> (w344:dbl[])
                  n169 = Initialize Array(w326, w347) -> (w343:dbl[])
                  n170 = Initialize Array(w325, w347) -> (w342:dbl[])
                  n171 = Initialize Array(w336, w347) -> (w361:dbl[])
                  n172 = Initialize Array(w333, w347) -> (w360:dbl[])
                  n173 = Initialize Array(w363, w347) -> (w368:dbl[])
                  n174 = Initialize Array(w362, w347) -> (w367:dbl[])
                  n175 = Bundle(w345, "sec"=w341) -> (w340:cluster{dbl[], "sec":dbl[]})  [unwired: 1 in]
                  n176 = Bundle(w344, "sec"=w341) -> (w339:cluster{dbl[], "sec":dbl[]})  [unwired: 1 in]
                  n177 = Bundle(w343, "sec"=w341) -> (w338:cluster{dbl[], "sec":dbl[]})  [unwired: 1 in]
                  n178 = Bundle(w342, "sec"=w341) -> (w337:cluster{dbl[], "sec":dbl[]})  [unwired: 1 in]
                  n179 = Bundle(w361, "sec"=w341) -> (w349:cluster{dbl[], "sec":dbl[]})  [unwired: 1 in]
                  n180 = Bundle(w360, "sec"=w341) -> (w348:cluster{dbl[], "sec":dbl[]})  [unwired: 1 in]
                  n181 = Bundle("sec"=w341, w368) -> (w372:cluster{"sec":dbl[], dbl[]})  [unwired: 1 in]
                  n182 = Bundle("sec"=w341, w367) -> (w366:cluster{"sec":dbl[], dbl[]})  [unwired: 1 in]
                  n183 = Build Array (concatenate)(w340, w339, w338, w337, w349, w348, w371, w372, w366) -> (→"Time trace":cluster{"sec":dbl[], "BM":dbl[]}[])
                }
                frame #1 {
                  n184 = local read "Save Time-trace"() -> (w481:bool)
                  n185 = local read "created path 2"() -> (w477:path)
                  n186 = local read "Save X-Y plot"() -> (w478:bool)
                  n187 = local read "created path"() -> (w479:path)
                  n188 = case shown="True" w478 {
                    tunnel: w480 -> [_ w488]
                    tunnel: w477 -> [_ w485]
                    frame False {
                    }
                    frame True {
                      n189 = Concatenate Strings("aoi" ("string"), w488, ".jpeg" ("string")) -> (w486:string)
                      n190 = invoke on="X-Y plot" class="XYGraph (strict)" method="Get Image"() -> ("image data"=w483:T7)  [unwired: 6 in, 5 out]
                      n191 = Build Path(base path=w485, name or relative path=w486) -> (appended path=w484:path)
                      n192 = call <vilib>:"Write JPEG File.vi"("image data"=w483, "path to JPEG file"=w484) -> ()  [unwired: 8 in, 2 out]
                    }
                  }
                  n193 = case shown="True" w481 {
                    tunnel: w480 -> [w489 w491]
                    tunnel: w479 -> [_ w494]
                    tunnel: [w489 w491] -> w476
                    frame False {
                    }
                    frame True {
                      n194 = Concatenate Strings("aoi" ("string"), w491, ".jpeg" ("string")) -> (w495:string)
                      n195 = invoke on="Time trace" class="XYGraph (strict)" method="Get Image"() -> ("image data"=w490:T7)  [unwired: 6 in, 5 out]
                      n196 = Build Path(base path=w494, name or relative path=w495) -> (appended path=w493:path)
                      n197 = call <vilib>:"Write JPEG File.vi"("image data"=w490, "path to JPEG file"=w493) -> ()  [unwired: 8 in, 2 out]
                    }
                  }
                  "aoi" <- w476
                }
              }
            }
          }
          "Xstd" <- w317
        }
        n198 = call <vilib>:"Histogram.vi"("X"=w302) -> ("Histogram Graph"=→"?":T3)  [unwired: 7 in, 3 out]
        n199 = Array Size(array=w302) -> (size(s)=w307:i32)
        "size(s)" <- w307
        n200 = local read "filename"() -> (w301:string)
        n201 = Insert Into Array(array=w299, index=0, new element=w301) -> (w298:string[])
      }
    }
    "filename" <- w25
  }
  "useful AOIs" <- w21
  "# of AOI" <- w20
  "ystd" <- w12
  "# of Frames" <- w13
  "xstd" <- w2
  n202 = call-poly <vilib>:"Mean.vi"("X"=w2) -> ("mean"=→"X":dbl)  [unwired: 1 out]
  n203 = call <vilib>:"Histogram.vi"("X"=w2) -> ("Histogram Graph"=→"?":T3)  [unwired: 7 in, 3 out]
  n204 = Transpose 2D Array(2D array=w4) -> (transposed array=→"Useful aoi number":string[][])
  n205 = Array Size(array=w2) -> (size(s)=w9:i32)
  "tt # 0f useful AOIs" <- w9
  "tt # of useful AOIs" <- w9
  n206 = Number To Decimal String(number=w9) -> (decimal integer string=w7:string)  [unwired: 1 in]
  n207 = Concatenate Strings("\\" ("string"), w7) -> (w6:string)
  n208 = case shown="True" "Save BM" {
    tunnel: w2 -> [_ w504]
    tunnel: w6 -> [_ w498]
    frame False {
    }
    frame True {
      n209 = local read "Folder path"() -> (w503:path)
      n210 = Path To String(path=w503) -> (string=w502:string)
      n211 = Concatenate Strings(w502, w498, ".txt" ("string")) -> (w501:string)
      n212 = String To Path(string=w501) -> (path=w500:path)
      n213 = call-poly <vilib>:"Write To Spreadsheet File.vi"("transpose? (no:F)"="Save to vertical data ?", "1D data"=w504, "file path (dialog if empty)"=w500) -> ()  [unwired: 5 in, 1 out]
    }
  }
  n214 = call-poly <vilib>:"Mean.vi"("X"=w12) -> ("mean"=→"Y":dbl)  [unwired: 1 out]
  n215 = Add Array Elements(numeric array=w20) -> (sum=w18:i32)
  "tt # of AOIs" <- w18
  n216 = Add Array Elements(numeric array=w21) -> (sum=w19:i32)
  n217 = Divide(x=w19, y=w18) -> (x/y=w17:dbl)
  n218 = Multiply(x=w17, y=100.0) -> (x*y=→"% of useful AOIs":dbl)
